vi "SVI-Common-NoErrorPrompt.vi"(7 "MsgIn":string) -> ()   [LabVIEW 2024]
panel:
  in  "Blank Button":bool
  out "Msg":string
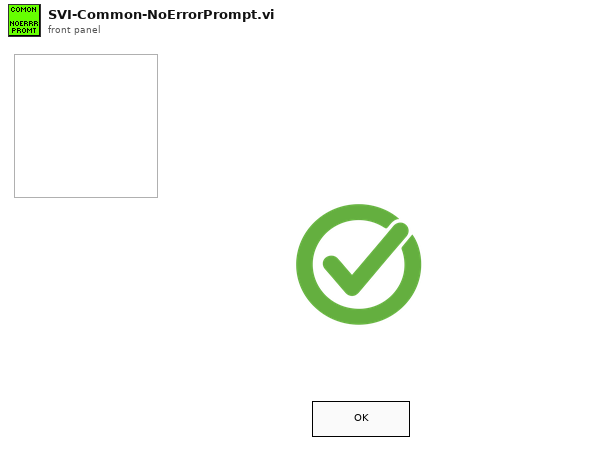
[diagram p1: front panel]
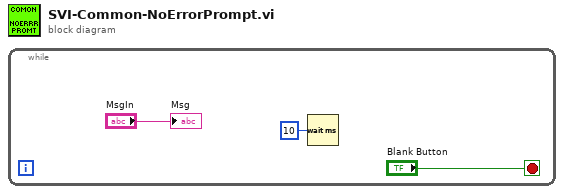
[diagram p0: block diagram]
diagram:
  n1 = while {
    stop <- "Blank Button" stop-if-true
    n2 = Wait (ms)(milliseconds to wait=u32 10) -> ()  [unwired: 1 out]
    "Msg" <- "MsgIn"
  }
